vi "GetValue.vi"(8 "error in":errorcluster, 11 "BooleanMeasure in":refnum<class "BooleanMeasure.lvclass">) -> (0 "error out":errorcluster, 2 "Value":bool, 3 "BooleanMeasure out":refnum<class "BooleanMeasure.lvclass">)   [LabVIEW 2021, in "ProligentXMLGenerator.lvlib" / "BooleanMeasure.lvclass"]
doc: "Defines the value acquired by the measure."
uses:
  BooleanMeasure.lvclass
  BooleanMeasure.lvclass/BooleanMeasure.ctl
  Base/Boolean/Boolean.lvclass
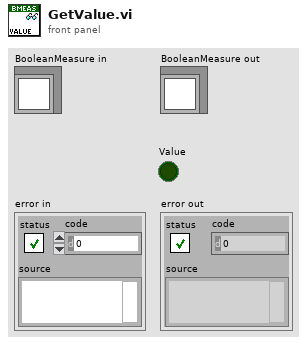
[diagram p1: front panel]
types:
  T1 = typedef "ProligentXMLGenerator.lvlib/BooleanMeasure.lvclass/Data.ctl" = cluster{"Value":refnum<class "Boolean.lvclass">}
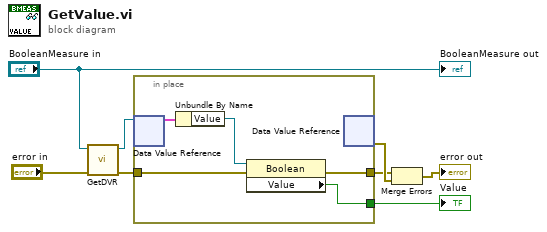
[diagram p0: block diagram]
diagram:
  n1 = call "GetDVR.vi"("error in"="error in", "BooleanMeasure"="BooleanMeasure in") -> ("error out"=w2:errorcluster, "DVRReference"=w7:refnum<data-value>)  [unwired: 8 in]
  n2 = in-place "In Place Element Structure" {
    in-place-border: [w9] -> w6
    in-place-border: w2 -> [w11]
    in-place-border: [w10] -> w1
    n3 = in-place-dvr #1(w7) -> (w13:T1)  [unwired: 1 out]
    n4 = Unbundle By Name(w13) -> ("Value"=w12:refnum<class "Boolean.lvclass">)
    n5 = property class="Boolean"(reference=w12, error in=w11) -> (error out=w10:errorcluster, "Value"=w9:bool)  [unwired: 1 out]
    n6 = in-place-dvr #1() -> (w8:errorcluster)  [unwired: 1 in, 1 out]
  }
  "Value" <- w6
  n7 = Merge Errors(w1, w8) -> (→"error out":errorcluster)
  "BooleanMeasure out" <- "BooleanMeasure in"
